vi "LabVIEW_OpenVINO_Demo.vi"() -> ()   [LabVIEW 2023]
uses:
  <vilib>/addons/VIRobotics/opencv_yiku/ctls/ColorConversionCodes.ctl
  <vilib>/addons/VIRobotics/opencv_yiku/ctls/Size.ctl
  <vilib>/addons/VIRobotics/opencv_yiku/Mat/Create_Mat_8UC3_Size.vi
  <vilib>/addons/VIRobotics/opencv_yiku/Cap/Cap.lvclass
  <vilib>/addons/VIRobotics/opencv_yiku/Mat/Mat_8U/Mat_8U.lvclass
  <vilib>/addons/VIRobotics/opencv_yiku/opencv_yiku.lvlib
panel:
  in  "Image Source":enum16{"USB Camera", "Video File"}(ring)=enum."Video File"
  in  "device_name":string="CPU"
  out "平均时间":dbl
  out "单帧时间":u32
  in  "stop":bool
  out "picture":picture
  in  "confidence":T1={"confThreshold"=0.3, "nms_threshold"=0.5}
  # "LabVIEW YOLOv8 Demo Based on OpenVINO"
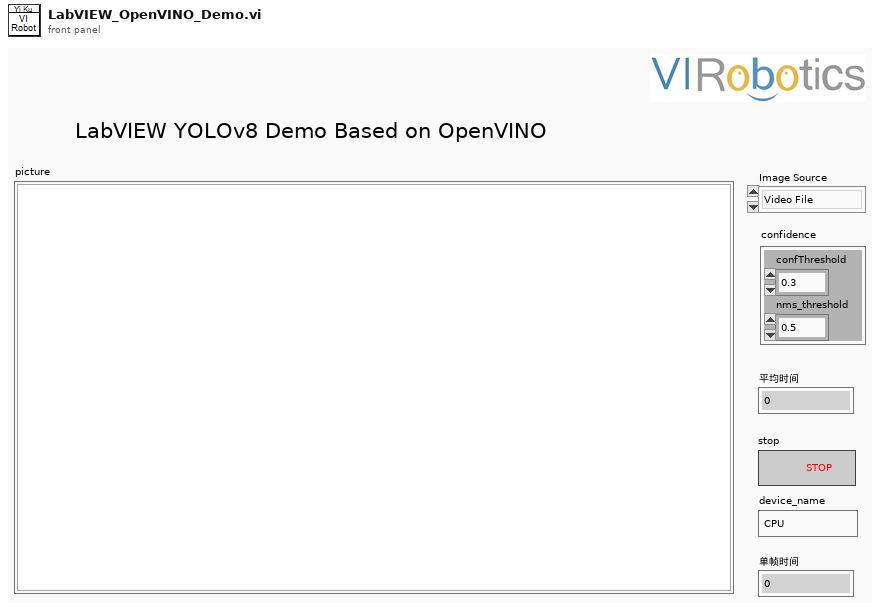
[diagram p1: front panel]
types:
  T1 = cluster{"confThreshold":sgl, "nms_threshold":sgl}
  T2 = typedef "opencv_yiku.lvlib/Size.ctl" = cluster{"x":i32, "y":i32}
  T3 = typedef "opencv_yiku.lvlib/ColorConversionCodes.ctl" = enum32{"COLOR_BGR2BGRA", "COLOR_BGRA2BGR", "COLOR_BGR2RGBA", "COLOR_RGBA2BGR", "COLOR_BGR2RGB", "COLOR_BGRA2RGBA", "COLOR_BGR2GRAY", "COLOR_RGB2GRAY", "COLOR_GRAY2BGR", "COLOR_GRAY2BGRA", "COLOR_BGRA2GRAY", "COLOR_RGBA2GRAY", "COLOR_BGR2BGR565", "COLOR_RGB2BGR565", "COLOR_BGR5652BGR", "COLOR_BGR5652RGB", "COLOR_BGRA2BGR565", "COLOR_RGBA2BGR565", "COLOR_BGR5652BGRA", "COLOR_BGR5652RGBA", "COLOR_GRAY2BGR565", "COLOR_BGR5652GRAY", "COLOR_BGR2BGR555", "COLOR_RGB2BGR555", "COLOR_BGR5552BGR", "COLOR_BGR5552RGB", "COLOR_BGRA2BGR555", "COLOR_RGBA2BGR555", "COLOR_BGR5552BGRA", "COLOR_BGR5552RGBA", "COLOR_GRAY2BGR555", "COLOR_BGR5552GRAY", "COLOR_BGR2XYZ", "COLOR_RGB2XYZ", "COLOR_XYZ2BGR", "COLOR_XYZ2RGB", "COLOR_BGR2YCrCb", "COLOR_RGB2YCrCb", "COLOR_YCrCb2BGR", "COLOR_YCrCb2RGB", "COLOR_BGR2HSV", "COLOR_RGB2HSV", "42", "43", "COLOR_BGR2Lab", "COLOR_RGB2Lab"}
  T4 = typedef "opencv_yiku.lvlib/Rect.ctl" = cluster{"x":i32, "y":i32, "width":i32, "height":i32}
  T5 = cluster{"boxes":T4[], "confidences":sgl[], "classes":i32[]}
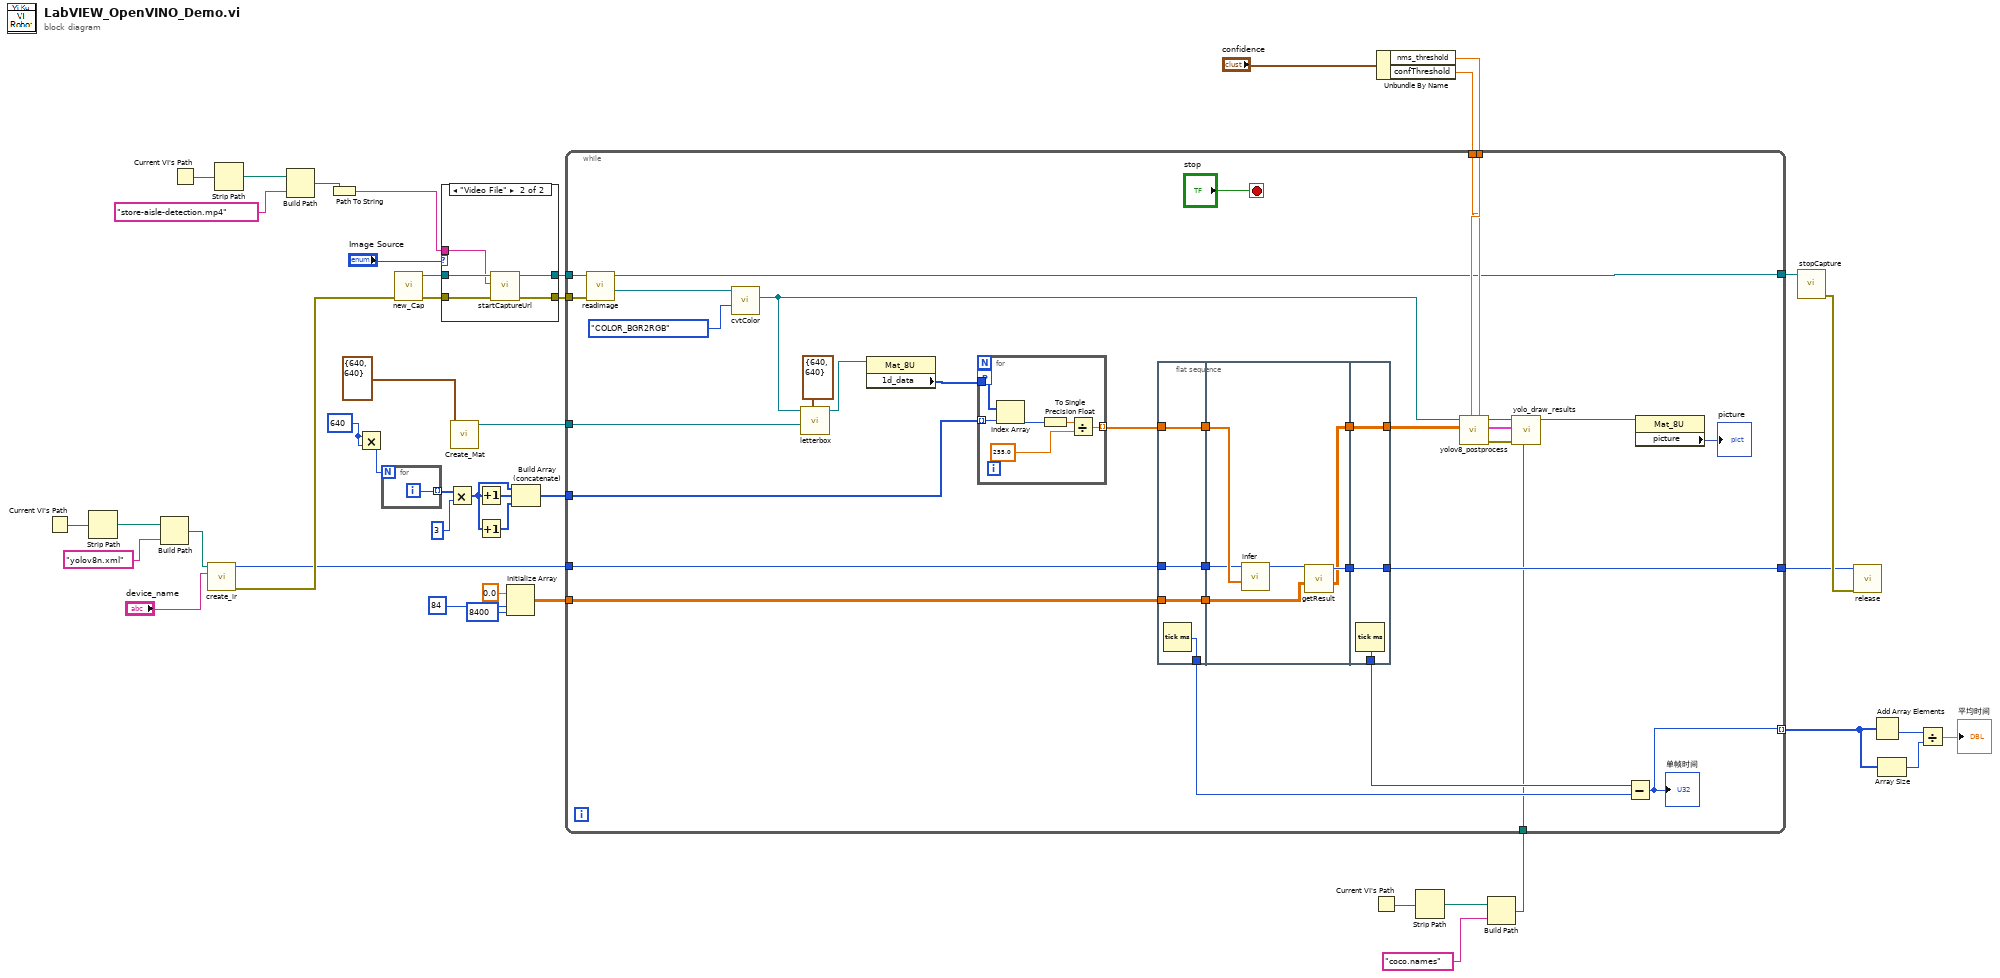
[diagram p0: block diagram]
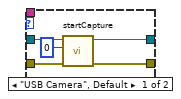
[diagram p2: hidden frame]
diagram:
  w35 = 640 ("x")
  n1 = Current VI's Path() -> (path=w4:path)
  n2 = Strip Path(path=w4) -> (stripped path=w3:path)  [unwired: 1 out]
  n3 = Build Path(base path=w3, name or relative path="yolov8n.xml") -> (appended path=w1:path)
  n4 = Current VI's Path() -> (path=w11:path)
  n5 = call "create_ir.vi"("device_name"="device_name", "xml_file"=w1) -> ("error out"=w18:errorcluster, "OvEngineStruct"=w15:u64)  [unwired: 8 in]
  n6 = Strip Path(path=w11) -> (stripped path=w12:path)  [unwired: 1 out]
  n7 = Build Path(base path=w12, name or relative path="store-aisle-detection.mp4") -> (appended path=w10:path)
  n8 = Path To String(path=w10) -> (string=w5:string)
  n9 = Multiply(x=w35, y=w35) -> (x*y=w34:i32)
  n10 = for {
    N: w34 -> [_]
    tunnel: [w46] -> w33 mode=indexing
    i -> [w46]
  }
  n11 = call <vilib>:"new_Cap.vi"("error in (no error)"=w18) -> ("error out"=w8:errorcluster, "Cap out"=w9:refnum<class "Cap.lvclass">)  [unwired: 9 in]
  n12 = case shown="\"Video File\"" "Image Source" {
    tunnel: [w51 w54] -> w28
    tunnel: w9 -> [w50 w56]
    tunnel: w8 -> [w49 w55]
    tunnel: [w48 w53] -> w7
    tunnel: w5 -> [_ w52]
    frame "USB Camera", Default {
      n13 = call <vilib>:"startCapture.vi"("error in (no error)"=w49, "cameraID"=0, "Cap in"=w50) -> ("error out"=w48:errorcluster, "Cap out"=w51:refnum<class "Cap.lvclass">)  [unwired: 7 in]
    }
    frame "Video File" {
      n14 = call-dynamic "startCaptureUrl.vi"("error in (no error)"=w55, "url"=w52, "Cap in"=w56) -> ("error out"=w53:errorcluster, "Cap out"=w54:refnum<class "Cap.lvclass">)  [unwired: 7 in]
    }
  }
  n15 = Multiply(x=w33, y=3) -> (x*y=w30:i32[])
  n16 = call-poly <vilib>:"Create_Mat.vi"("Size"=cluster{"x":i32, "y":i32} {"x"=640, "y"=640}) -> ("Mat_8U_out"=w36:refnum<class "Mat_8U.lvclass">)  [unwired: 9 in, 1 out]
  n17 = Increment(x=w30) -> (x+1=w31:i32[])
  n18 = Increment(x=w30) -> (x+1=w29:i32[])
  n19 = Initialize Array(sgl 0.0 ("element"), 84 ("dimension size"), 8400 ("dimension size")) -> (w41:sgl[][])
  n20 = Build Array (concatenate)(w30, w31, w29) -> (w24:i32[])
  n21 = Current VI's Path() -> (path=w22:path)
  n22 = Unbundle By Name("confidence") -> ("nms_threshold"=w43:sgl, "confThreshold"=w42:sgl)
  n23 = Strip Path(path=w22) -> (stripped path=w21:path)  [unwired: 1 out]
  n24 = Build Path(base path=w21, name or relative path="coco.names") -> (appended path=w19:path)
  n25 = while {
    tunnel: w41 -> [w88]
    tunnel: w43 -> [w85]
    tunnel: w42 -> [w84]
    tunnel: [w83] -> w37 mode=indexing
    tunnel: w36 -> [w82]
    tunnel: [w81] -> w14
    tunnel: w28 -> [w80]
    tunnel: [w78] -> w27
    tunnel: w24 -> [w77]
    tunnel: w19 -> [w61]
    tunnel: w15 -> [w59]
    tunnel: w7 -> [w57]
    stop <- "stop" stop-if-true
    n26 = call <vilib>:"readImage.vi"("error in (no error)"=w57, "Cap in"=w80) -> ("Mat out"=w79:refnum<class "Mat_8U.lvclass">, "Cap out"=w78:refnum<class "Cap.lvclass">)  [unwired: 7 in, 1 out]
    n27 = call <vilib>:"cvtColor.vi"("dstCn"=ColorConversionCodes."COLOR_BGR2RGB", "src"=w79) -> ("dst out"=w70:refnum<class "Mat_8U.lvclass">)  [unwired: 7 in, 2 out]
    n28 = call "letterbox.vi"("Size"=T2 {"x"=640, "y"=640}, "resized"=w82, "image"=w70) -> ("resized out"=w75:refnum<class "Mat_8U.lvclass">)  [unwired: 7 in, 1 out]
    n29 = property class="Mat_8U"(reference=w75) -> ("1d_data"=w76:u8[])  [unwired: 1 in, 2 out]
    n30 = for {
      tunnel: w76 -> [w108]
      tunnel: [w107] -> w68 mode=indexing
      workers-P: _ -> [_]
      tunnel: w77 -> [w103] mode=indexing
      n31 = Index Array(array=w108, index=w103) -> (element=w105:u8)
      n32 = To Single Precision Float(number=w105) -> (single precision float=w104:sgl)
      n33 = Divide(x=w104, y=sgl 255.0) -> (x/y=w107:sgl)
    }
    n34 = flat-sequence {
      tunnel: w68 -> [w92]
      tunnel: w88 -> [w93]
      tunnel: [w93] -> w67
      tunnel: [w92] -> w66
      tunnel: [w91] -> w62
      tunnel: w59 -> [w90]
      tunnel: [w90] -> w58
      tunnel: w67 -> [w99]
      tunnel: w66 -> [w96]
      tunnel: [w98] -> w65
      tunnel: [w97] -> w64
      tunnel: w58 -> [w95]
      tunnel: [w101] -> w60
      tunnel: [w102] -> w81
      tunnel: w65 -> [w102]
      tunnel: w64 -> [w101]
      tunnel: [w100] -> w63
      frame #0 {
        n35 = Tick Count (ms)() -> (millisecond timer value=w91:u32)
      }
      frame #1 {
        n36 = call "infer.vi"("data"=w96, "InferEngineStruct"=w95) -> ("InferEngineStruct out"=w94:u64)  [unwired: 8 in, 1 out]
        n37 = call "getResult.vi"("data_shape"=w99, "InferEngineStruct"=w94) -> ("data out"=w97:sgl[][], "InferEngineStruct out"=w98:u64)  [unwired: 7 in, 1 out]
      }
      frame #2 {
        n38 = Tick Count (ms)() -> (millisecond timer value=w100:u32)
      }
    }
    n39 = call "yolov8_postprocess.vi"("nms_threshold"=w85, "confThreshold"=w84, "2d_data"=w60, "image"=w70) -> ("error out"=w72:errorcluster, "results"=w71:T5, "reference out"=w73:refnum<class "Mat_8U.lvclass">)  [unwired: 5 in]
    n40 = call "yolo_draw_results.vi"("coco_names"=w61, "error in (no error)"=w72, "results"=w71, "image"=w73) -> ("img out"=w86:refnum<class "Mat_8U.lvclass">)  [unwired: 6 in, 1 out]
    n41 = Subtract(x=w63, y=w62) -> (x-y=w83:u32)
    "单帧时间" <- w83
    n42 = property class="Mat_8U"(reference=w86) -> ("picture"=→"picture":picture)  [unwired: 1 in, 2 out]
  }
  n43 = call <vilib>:"stopCapture.vi"("Cap in"=w27) -> ("error out"=w26:errorcluster)  [unwired: 10 in]
  n44 = call "release.vi"("error in (no error)"=w26, "InferEngineStruct"=w14) -> ()  [unwired: 9 in, 1 out]
  n45 = Add Array Elements(numeric array=w37) -> (sum=w40:u32)
  n46 = Array Size(array=w37) -> (size(s)=w39:i32)
  n47 = Divide(x=w40, y=w39) -> (x/y=→"平均时间":dbl)
